vi "Unflatten Attr Priv.vi"(5 "Data Types Dict":variant, 6 "After First Tag String":string, 7 "Parsed Header":T1, 8 "error in":errorcluster, 10 "Parent ID (empty)":string, 11 "Tree Dict":variant) -> (0 "error out":errorcluster, 3 "Tree Dictionary Out":variant, 4 "After First Tag String":string)   [LabVIEW 2017, in "Tree API.lvlib" / "Tree.lvclass"]
uses:
  Tree.lvclass
  <vilib>/ErrorRing/Error Ring.xnode
  Tree Data/Tree Data.lvclass
  <vilib>/Utility/error.llb/Error Cluster From Error Code.vi
  Parsed Header.ctl
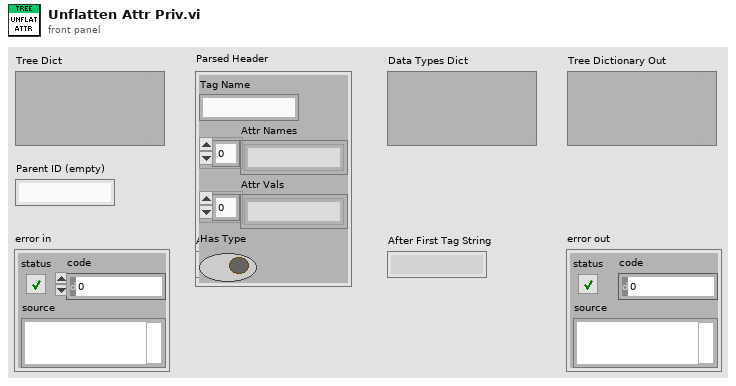
[diagram p1: front panel]
types:
  T1 = typedef "Tree API.lvlib/Tree.lvclass/Parsed Header.ctl" = cluster{"Tag Name":string, "Attr Names":string[], "Attr Vals":string[], "Has Type":bool}
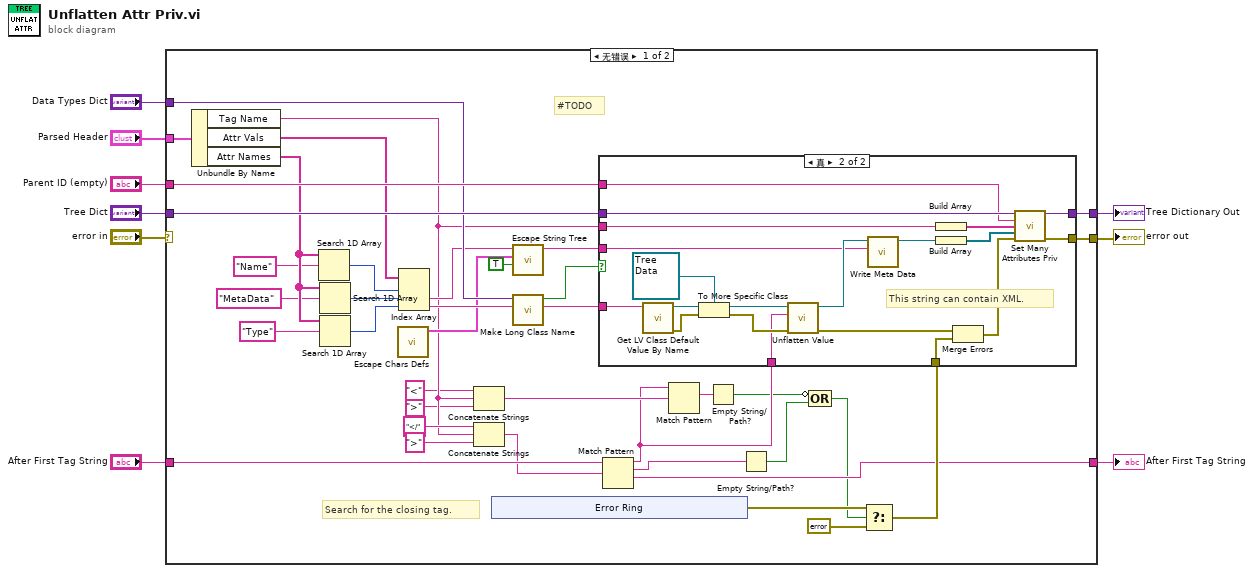
[diagram p0: block diagram]
diagram:
  n1 = case shown="无错误" "error in" {
    selector: "error in" -> [_ w78]
    tunnel: "Data Types Dict" -> [w27 _]
    tunnel: "Parent ID (empty)" -> [w45 _]
    tunnel: "Tree Dict" -> [w44 w77]
    tunnel: [w43 w78] -> w6
    tunnel: [w42 w77] -> w5
    tunnel: [w41 w76] -> w4
    tunnel: "After First Tag String" -> [w39 w76]
    tunnel: "Parsed Header" -> [w35 _]
    frame No Error {
      # "Search for the closing tag."
      # "#TODO"
      n2 = Unbundle By Name(w35) -> ("Tag Name"=w18:string, "Attr Vals"=w37:string[], "Attr Names"=w36:string[])
      n3 = Search 1D Array(1D array=w36, element="Name") -> (index of element=w34:i32)  [unwired: 1 in]
      n4 = Search 1D Array(1D array=w36, element="MetaData") -> (index of element=w30:i32)  [unwired: 1 in]
      n5 = Search 1D Array(1D array=w36, element="Type") -> (index of element=w32:i32)  [unwired: 1 in]
      n6 = call "Escape Chars Defs.vi"() -> ("Escapes"=w23:cluster{"String":string, "Escape":string}[])  [unwired: 11 in]
      n7 = Index Array(array=w37, index #1=w34, index #2=w30, index #3=w32) -> (element #2=w25:string, element #3=w26:string)  [unwired: 1 out]
      n8 = Concatenate Strings("<" ("string"), w18, ">" ("string")) -> (w15:string)
      n9 = Concatenate Strings("</" ("string"), w18, ">" ("string")) -> (w19:string)
      n10 = xnode "Error Ring"() -> ("错误输出"=w38:errorcluster)
      n11 = call "Escape String Tree.vi"("Reverse? (False)"=TRUE, "Escapes"=w23, "String In"=w25) -> ("String Out"=w24:string)  [unwired: 8 in]
      n12 = call "Make Long Class Name.vi"("Short Class Name"=w26, "Data Types Dict"=w27) -> ("Long Class Name"=w28:string, "Found"=w47:bool)  [unwired: 8 in]
      n13 = Match Pattern(string=w39, regular expression=w19) -> (before substring=w14:string, match substring=w40:string, after substring=w41:string)  [unwired: 1 in, 1 out]
      n14 = Match Pattern(string=w14, regular expression=w15) -> (match substring=w13:string)  [unwired: 1 in, 3 out]
      n15 = Empty String/Path?(string/path=w13) -> (empty?=w12:bool)
      n16 = Empty String/Path?(string/path=w40) -> (empty?=w11:bool)
      n17 = Compound Arithmetic op=OR(invert w12, w11) -> (w10:bool)
      n18 = Select(t=w38, s=w10, f=errorcluster {"status"=FALSE, "code"=0, "source"=""}) -> (s? t:f=w46:errorcluster)
      n19 = case shown="真" w47 {
        tunnel: w24 -> [_ w64]
        tunnel: w14 -> [_ w63]
        tunnel: [w49 w62] -> w42
        tunnel: [w50 w61] -> w43
        tunnel: w44 -> [w49 w60]
        tunnel: w45 -> [_ w59]
        tunnel: w18 -> [_ w58]
        tunnel: w46 -> [w50 w52]
        tunnel: w28 -> [_ w54]
        frame False {
        }
        frame True {
          # "This string can contain XML."
          n20 = call <vilib>:"Get LV Class Default Value By Name.vi"("class name"=w54) -> ("error out"=w67:errorcluster, "object"=w70:refnum<class>)  [unwired: 9 in]
          n21 = To More Specific Class(target class=refnum<class "Tree Data.lvclass"> refnum ("Tree Data In"), reference=w70, error in=w67) -> (specific class reference=w68:refnum<class "Tree Data.lvclass">, error out=w66:errorcluster)
          n22 = call-dynamic "Unflatten Value.vi"("Error In"=w66, "Value"=w63, "Tree Data In"=w68) -> ("Error Out"=w53:errorcluster, "Tree Data Out"=w65:refnum<class "Tree Data.lvclass">)  [unwired: 7 in]
          n23 = call "Write Meta Data.vi"("Meta Data"=w64, "Tree Data In"=w65) -> ("Tree Data Out"=w56:refnum<class "Tree Data.lvclass">)  [unwired: 9 in]
          n24 = Build Array(w58) -> (w57:string[])
          n25 = Build Array(w56) -> (w55:refnum<class "Tree Data.lvclass">[])
          n26 = Merge Errors(w53, w52) -> (w51:errorcluster)
          n27 = call "Set Many Attributes Priv.vi"("Tree Dictionary Out"=w60, "Unique ID"=w59, "Name"=w57, "Data"=w55, "error in"=w51) -> ("Tree Dictionary Out"=w62:variant, "error out"=w61:errorcluster)  [unwired: 8 in, 1 out]
        }
      }
    }
    frame Error {
    }
  }
  "error out" <- w6
  "Tree Dictionary Out" <- w5
  "After First Tag String" <- w4
